vi "copmuter t0.vi"(9 "time":dbl, 10 "nchanelSize":i32=8192, 11 "t0 in":timestamp) -> (2 "t0 out":timestamp)   [LabVIEW 2009]
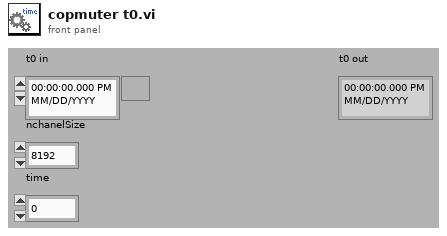
[diagram p1: front panel]
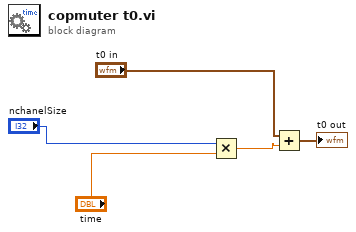
[diagram p0: block diagram]
diagram:
  n1 = Multiply(x="nchanelSize", y="time") -> (x*y=w1:dbl)
  n2 = Add(x="t0 in", y=w1) -> (x+y=→"t0 out":timestamp)
